vi "RingQueue.vi"(0 "Prev Solenoid Data":bool, 1 "Curr Solenoid Data":bool, 3 "Program control":bool, 7 "RingQueue":refnum<vi>) -> ()   [LabVIEW 2016]
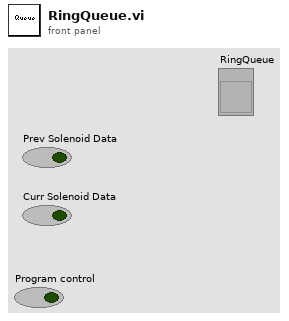
[diagram p1: front panel]
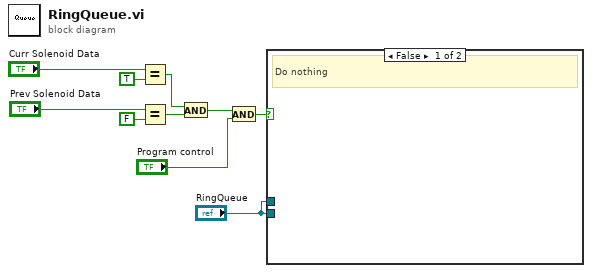
[diagram p0: block diagram]
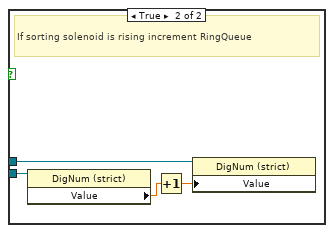
[diagram p2: hidden frame]
diagram:
  n1 = Equal?(x="Curr Solenoid Data", y=TRUE) -> (x = y?=w5:bool)
  n2 = Equal?(x="Prev Solenoid Data", y=FALSE) -> (x = y?=w4:bool)
  n3 = And(x=w5, y=w4) -> (x .and. y?=w3:bool)
  n4 = And(x=w3, y="Program control") -> (x .and. y?=w2:bool)
  n5 = case shown="False" w2 {
    tunnel: "RingQueue" -> [_ w12]
    tunnel: "RingQueue" -> [_ w11]
    frame False {
      # "Do nothing"
    }
    frame True {
      # "If sorting solenoid is rising increment RingQueue"
      n6 = property class="DigNum (strict)"(reference=w12) -> ("Value"=w14:dbl)  [unwired: 1 in, 2 out]
      n7 = Increment(x=w14) -> (x+1=w13:dbl)
      n8 = property class="DigNum (strict)"(reference=w11, "Value"=w13) -> ()  [unwired: 1 in, 2 out]
    }
  }
